vi "Read Multi Eval Meas Trace Power Dynamics Results.vi"(8 "error in (no error)":errorcluster {"code" format="%.0x"}, 9 "Result Type (Current)":i32(ring) items=["Current"=0, "Average"=1, "Maximum"=4], 10 "Instance (1)":T1=1, 11 "VISA resource name":refnum<visa-resource-name>) -> (0 "error out":errorcluster {"code" format="%.0x"}, 1 "Results":dbl[](array[numeric]) format="%^.3e", 2 "Reliability":i32, 3 "VISA resource name out":refnum<visa-resource-name>)   [LabVIEW 2020, in "Rohde&Schwarz CMWXP NR FR1 Measurement.lvlib"]
doc: "Return the values of the power dynamics traces. Each value is sampled with 48 Ts, corresponding to 1.5625 us. The results of the current, average and maximum traces can be retrieved.\n\nAttributes:\nRSCMWXPNRFR1M_ATTR_READ_MULTI_MEAS_EVAL_TRACE_POWER_DYNAMICS_CURRENT_RESULTS\nRSCMWXPNRFR1M_ATTR_READ_MULTI_MEAS_EVAL_TRACE_POWER_DYNAMICS_AVERAGE_RESULTS\nRSCMWXPNRFR1M_ATTR_READ_MULTI_MEAS_EVAL_TRACE_POWER_DYNAMICS_MAXIMUM_RESULTS\n\nRemote-control commands:\nREAD:NRSub:MEAS<i>:MEValuation:TRACe:PDYNamics:CURRent?\nREAD:NRSub:MEAS<i>:MEValuation:TRACe:PDYNamics:AVERage?\nREAD:NRSub:MEAS<i>:MEValuation:TRACe:PDYNamics:MAXimum?"
uses:
  <instrlib>/Rohde&Schwarz CMWXP NR FR1 Measurement/Rohde&Schwarz CMWXP NR FR1 Measurement.lvlib
  <instrlib>/Rohde&Schwarz CMWXP NR FR1 Measurement/Private/_Instance.ctl
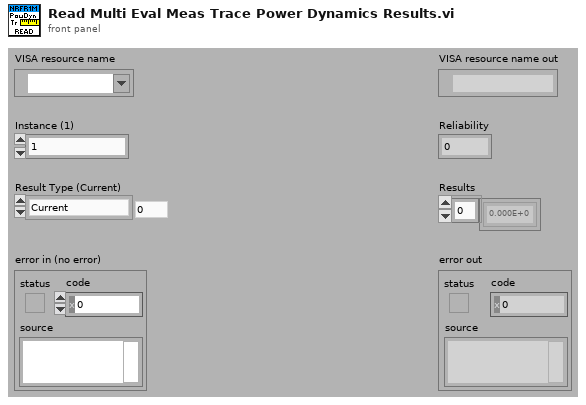
[diagram p1: front panel]
types:
  T1 = typedef "Rohde&Schwarz CMWXP NR FR1 Measurement.lvlib/_Instance.ctl" = i32
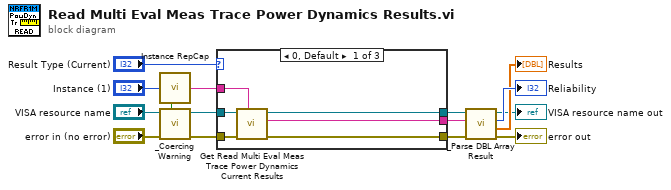
[diagram p0: block diagram]
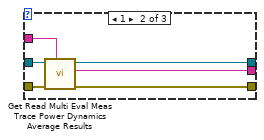
[diagram p2: hidden frame]
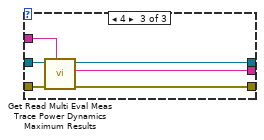
[diagram p3: hidden frame]
diagram:
  n1 = call <instrlib>:"Instance RepCap.vi"("Instance In"="Instance (1)") -> ("In Range?"=w12:bool, "RepCap Identifier Out"=w9:string)  [unwired: 1 in]
  n2 = call <instrlib>:"_Coercing Warning.vi"("In Range?"=w12, "error in (no error)"="error in (no error)", "VISA resource name"="VISA resource name") -> ("error out"=w10:errorcluster, "VISA resource name out"=w11:refnum<visa-resource-name>)  [unwired: 7 in]
  n3 = case shown="0, Default" "Result Type (Current)" {
    tunnel: w11 -> [w21 w27 w33]
    tunnel: w10 -> [w20 w26 w32]
    tunnel: w9 -> [w19 w25 w31]
    tunnel: [w18 w24 w30] -> w5
    tunnel: [w17 w23 w29] -> w6
    tunnel: [w16 w22 w28] -> w7
    frame 0, Default {
      n4 = call "Get Read Multi Eval Meas Trace Power Dynamics Current Results"("Repeated Capabilities"=w19, "error in (no error)"=w20, "instrument handle"=w21) -> ("error out"=w16:errorcluster, "Read Multi Eval Meas Trace Power Dynamics Current Results"=w17:string, "instrument handle out"=w18:refnum<visa-resource-name>)  [unwired: 6 in]
    }
    frame 1 {
      n5 = call "Get Read Multi Eval Meas Trace Power Dynamics Average Results"("Repeated Capabilities"=w25, "error in (no error)"=w26, "instrument handle"=w27) -> ("error out"=w22:errorcluster, "Read Multi Eval Meas Trace Power Dynamics Average Results"=w23:string, "instrument handle out"=w24:refnum<visa-resource-name>)  [unwired: 6 in]
    }
    frame 4 {
      n6 = call "Get Read Multi Eval Meas Trace Power Dynamics Maximum Results"("Repeated Capabilities"=w31, "error in (no error)"=w32, "instrument handle"=w33) -> ("error out"=w28:errorcluster, "Read Multi Eval Meas Trace Power Dynamics Maximum Results"=w29:string, "instrument handle out"=w30:refnum<visa-resource-name>)  [unwired: 6 in]
    }
  }
  n7 = call <instrlib>:"_Parse DBL Array Result.vi"("error in (no error)"=w7, "Input String"=w6, "VISA resource name"=w5) -> ("error out"=→"error out":errorcluster, "Results"=→"Results":dbl[], "Reliability"=→"Reliability":i32, "VISA resource name out"=→"VISA resource name out":refnum<visa-resource-name>)  [unwired: 5 in]
